vi "Position module.vi"(8 "error in (no error)":errorcluster) -> (0 "error out":errorcluster)   [LabVIEW 2016]
uses:
  General/Controls/data modes.ctl
  DAQ/Controls/DAQ queue.ctl
  DAQ/Controls/Queue states.ctl
  General/Controls/Queue modes.ctl
  Controls/Actuator fgv modes.ctl
  General/Controls/staus modes.ctl
  Controls/Command cluster.ctl
  Controls/Command list.ctl
  General/Controls/State control cluster.ctl
  General/Controls/States.ctl
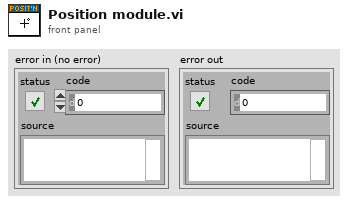
[diagram p1: front panel]
types:
  T1 = typedef "Queue modes.ctl" = enum16{"Initialise", "Destroy", "Get"}
  T2 = typedef "DAQ queue.ctl" = cluster{"Sate":T3, "Data":variant}
  T3 = typedef "Queue states.ctl" = enum16{"Shutdown", "Save data", "Record", "Read", "Setup", "Zero", "Connect", "Initialise"}
  T4 = typedef "data modes.ctl" = enum16{"Initalise", "Status", "Process", "Add load", "Add position"}
  T5 = cluster{"seconds since 1Jan1904":timestamp, "Numeric 2":dbl}[]
  T6 = typedef "References.ctl" = cluster{"Tab Control":refnum<vi>, "Logo 1":refnum<vi>, "Logo 2":refnum<vi>, "Connect Actuator":refnum<vi>, "LIVE DATA":refnum<vi>, "Speed":refnum<vi>, "Home position":refnum<vi>, "Limit position":refnum<vi>, "Trigger":refnum<vi>, "Current position":refnum<vi>, "Connect Camera":refnum<vi>, "TEST DATA":refnum<vi>, "LIVE DATA Force":refnum<vi>, "Connect DAQ":refnum<vi>, "Initialised":refnum<vi>, "Test":refnum<vi>}
  T7 = typedef "UEs.ctl" = cluster{"Read position":refnum<user-event>, "Check home":refnum<user-event>, "Record":refnum<user-event>, "Abort controller":refnum<user-event>, "Remote test":refnum<user-event>, "Test setup":refnum<user-event>, "Conditional wait":refnum<user-event>, "Abort move":refnum<user-event>, "Wait done":refnum<user-event>, "Send trigger":refnum<user-event>, "Initalising":refnum<user-event>, "Initalisation complete":refnum<user-event>}
  T8 = typedef "staus modes.ctl" = enum16{"Status", "Testing", "Webcam", "DAQ", "Actuator", "Initialise"}
  T9 = typedef "Actuator fgv modes.ctl" = enum16{"Initalise", "COM", "Limit", "Speed", "Home", "Get"}
  T10 = typedef "State control cluster.ctl" = cluster{"State":T11, "Data":variant}
  T11 = typedef "States.ctl" = enum16{"Initialise", "Actuator connection", "Get info", "Send command", "Load method", "Run method", "Save test", "Setup", "Shutdown"}
  T12 = typedef "Command cluster.ctl" = cluster{"Command":T13, "data":variant}
  T13 = typedef "Command list.ctl" = enum16{"", "£nabort", "getaxisno", "£getserialno", "£nidentify", "&&£setnlimit", "&£nm", "&£snv", "&£speed", "£np", "£ncal"}
  T14 = typedef "Default settings.ctl" = cluster{"COM port":refnum<visa-resource-name>, "Home pos":dbl, "Speed":dbl, "Limit stop":dbl}
  T15 = cluster{"seconds since 1Jan1904":timestamp, "Numeric 2":dbl}
  T16 = typedef "Test settings.ctl" = cluster{"Speed (mm/s)":dbl, "Position limit":bool, "Position limit (mm)":dbl, "Load limit":bool, "Load limit (N)":dbl, "No. of repeats":u16, "Test identifier":string, "Time wait":bool, "Wait time (s)":dbl, "Trigger wait":bool, "Send trigger":bool, "Test notes":string, "Snap intervals":bool, "Time interval (s)":dbl}
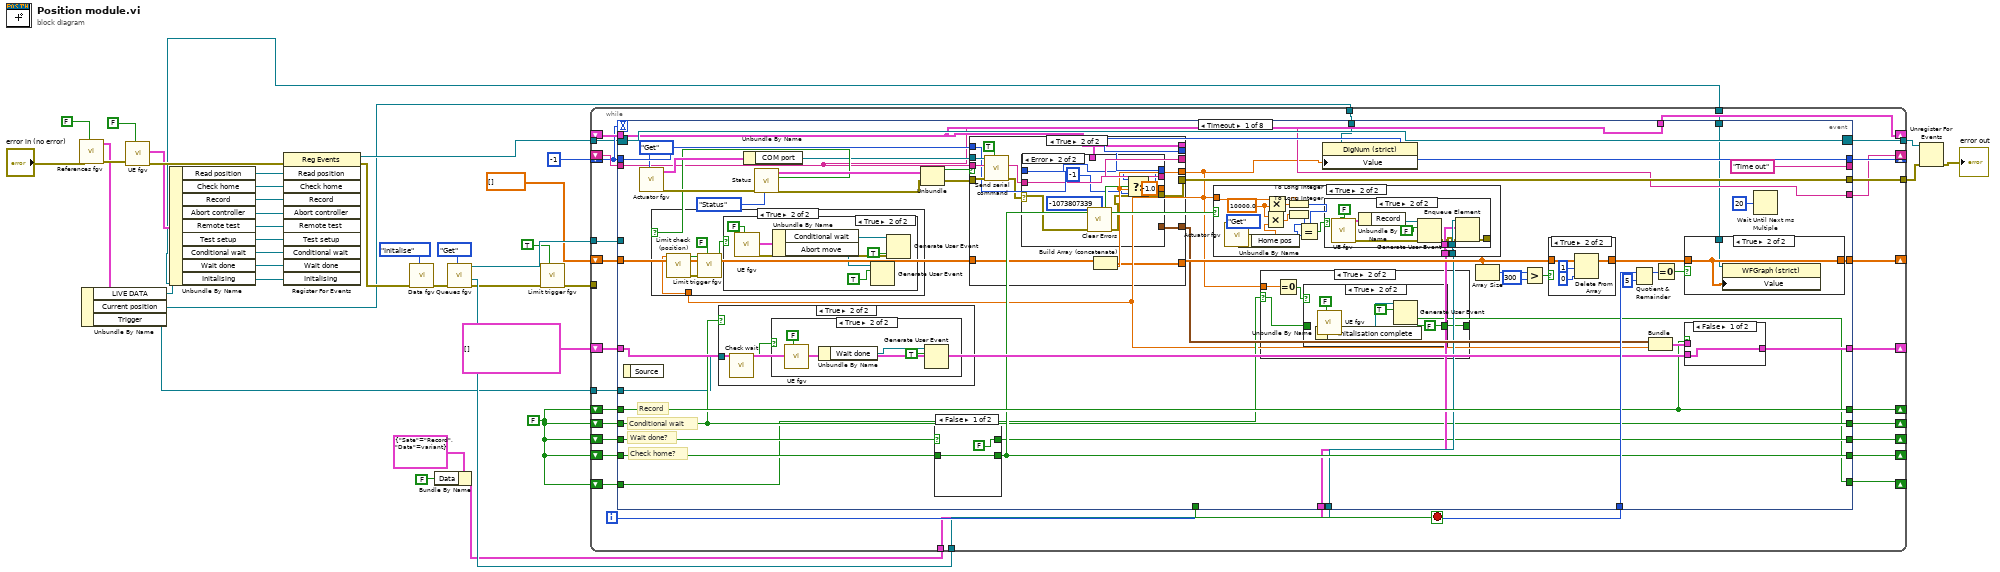
[diagram p0: block diagram]
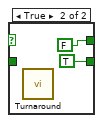
[diagram p10: hidden frame]
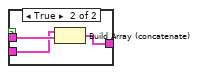
[diagram p11: hidden frame]
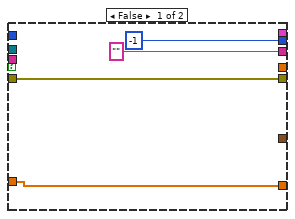
[diagram p14: hidden frame]
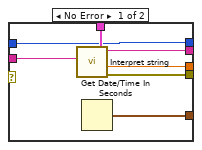
[diagram p15: hidden frame]
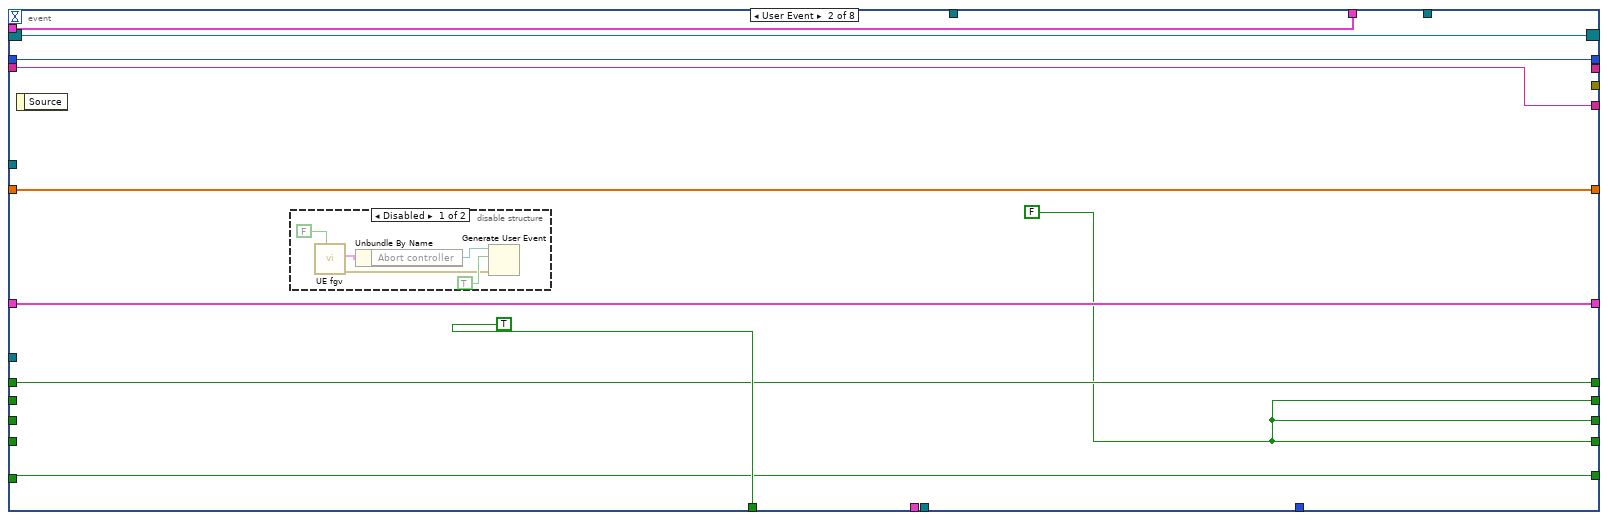
[diagram p16: hidden frame]
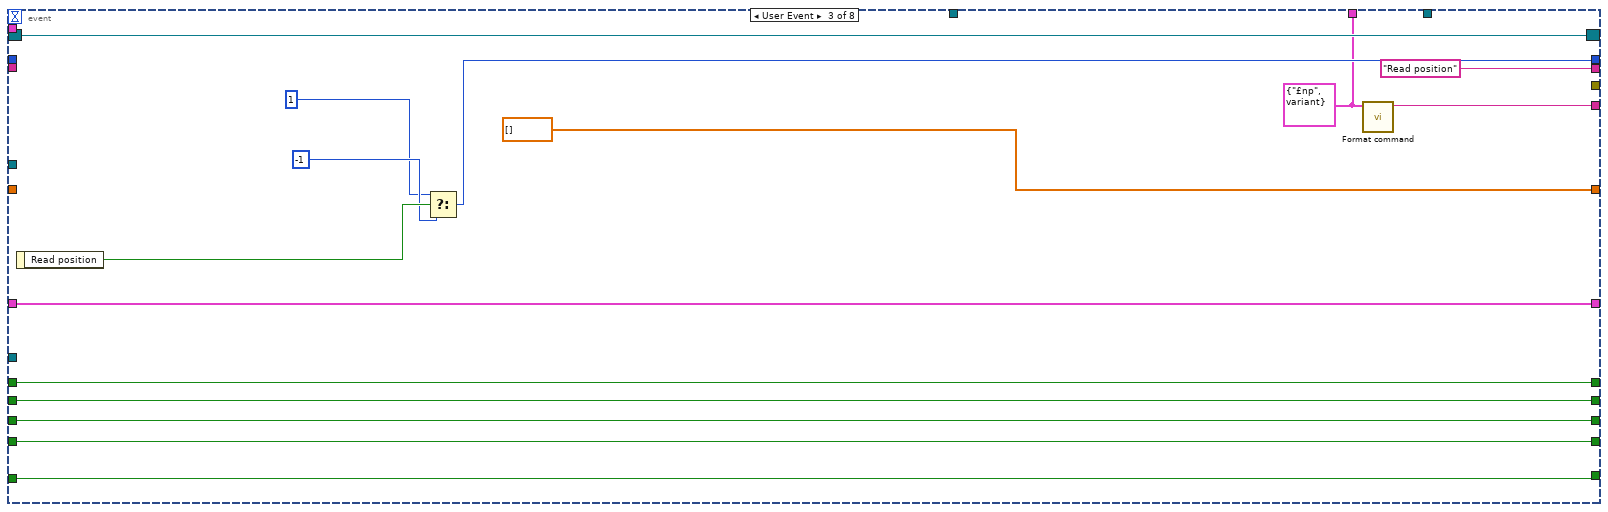
[diagram p18: hidden frame]
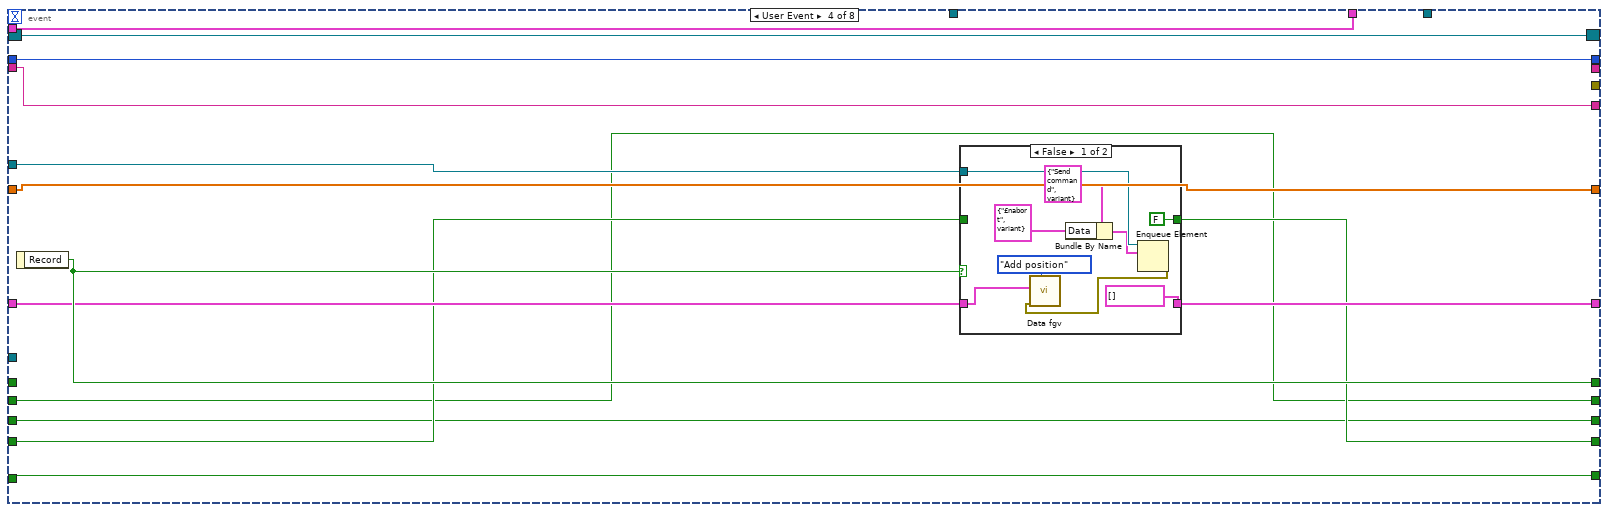
[diagram p19: hidden frame]
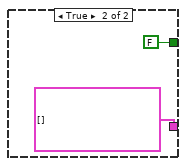
[diagram p20: hidden frame]
diagram:
  w1 = FALSE ("Record")
  n1 = call "References fgv.vi"("Set?"=FALSE, "error in (no error)"="error in (no error)") -> ("error out"=w8:errorcluster, "Cluster"=w6:T6)  [unwired: 8 in]
  n2 = Unbundle By Name(w6) -> ("LIVE DATA"=w3:refnum<vi>, "Current position"=w4:refnum<vi>, "Trigger"=w5:refnum<vi>)
  n3 = call "UE fgv.vi"("Set?"=FALSE, "error in (no error)"=w8) -> ("error out"=w33:errorcluster, "UEs"=w30:T7)  [unwired: 7 in, 1 out]
  n4 = Unbundle By Name(w30) -> ("Read position"=w19:refnum<user-event>, "Check home"=w20:refnum<user-event>, "Record"=w21:refnum<user-event>, "Abort controller"=w22:refnum<user-event>, "Remote test"=w23:refnum<user-event>, "Test setup"=w24:refnum<user-event>, "Conditional wait"=w26:refnum<user-event>, "Wait done"=w27:refnum<user-event>, "Initalising"=w2:refnum<user-event>)
  n5 = register-events(error in=w33, w19, w20, w21, w22, w23, w24, w26, w27, w2) -> (reference out=w25:refnum<event-registration>, error out=w32:errorcluster)  [unwired: 1 in]
  n6 = call "Data fgv.vi"("Modes"=data_modes."Initalise", "error in (no error)"=w32) -> ("error out"=w11:errorcluster)  [unwired: 5 in, 4 out]
  n7 = Bundle By Name(cluster=T2 {"Sate"=enum."Record", "Data"=variant} ("element"), "Data"=FALSE) -> (w18:T2)
  n8 = call "Queues fgv.vi"("Modes"=Queue_modes."Get", "error in (no error)"=w11) -> ("error in (no error) 2"=w10:errorcluster, "DAQ"=w39:refnum<queue>, "Ivium"=w38:refnum<queue>)  [unwired: 6 in, 1 out]
  n9 = call "Limit trigger fgv.vi"("Reset"=TRUE, "error in (no error)"=w10) -> ("error out"=w28:errorcluster)  [unwired: 8 in, 1 out]
  n10 = while {
    tunnel: [w69] -> w35
    tunnel: w25 -> [w53]
    shift-right: [w67] -> _
    shift-left: -1 -> [w66]
    shift-right: [w64] -> _
    shift-left: dbl[] [] -> [w65]
    shift-right: [w62] -> _
    shift-left: w1 -> [w61]
    shift-right: [w59] -> _
    shift-left: T5 [] -> [w60]
    tunnel: w39 -> [w58]
    tunnel: w18 -> [w57]
    tunnel: w38 -> [w56]
    shift-right: [w54] -> _
    shift-left: w1 -> [w55]
    shift-right: [w51] -> _
    shift-left: w1 -> [w52]
    shift-right: [w49] -> _
    shift-left: w1 -> [w50]
    tunnel: [w48] -> _
    tunnel: w28 -> [w48]
    tunnel: w5 -> [w47]
    tunnel: [w46] -> w34
    shift-right: [w45] -> _
    shift-left: _ -> [w70]
    shift-right: [w44] -> _
    shift-left: _ -> [w71]
    tunnel: w4 -> [w43]
    tunnel: w3 -> [w42]
    shift-right: [w40] -> _
    shift-left: w1 -> [w41]
    i -> [w63]
    stop <- w68 stop-if-true
    n11 = event shown="[0] Timeout" {
      selector: w53 -> [w116 w227 w244 w261 w280 w298 w315 w326]
      dyn-events: [w116 w227 w244 w261 w280 w298 w315 w326] -> w46
      timeout: w66 -> [_ _ _ _ _ _ _ _]
      tunnel: w71 -> [w77 w220 _ w250 w275 w286 w309 w322]
      tunnel: w70 -> [w78 w221 _ w251 w276 w287 w310 w323]
      tunnel: [w117 _ _ _ _ _ _ _] -> w69
      tunnel: [_ TRUE _ _ _ _ _ _] -> w68
      tunnel: [w113 w226 w245 w262 w281 w299 w316 w327] -> w67
      tunnel: w66 -> [w114 w226 _ w262 w281 w299 w316 w327]
      tunnel: w65 -> [w107 w225 _ w257 w282 w300 w317 w328]
      tunnel: [w84 w225 dbl[] [] w257 w282 w300 w317 w328] -> w64
      tunnel: w63 -> [w102 _ _ _ _ _ _ _]
      tunnel: [w94 w223 w241 w260 w279 w297 w314 w325] -> w62
      tunnel: w61 -> [w94 w223 w241 _ w279 w297 w314 w325]
      tunnel: w60 -> [w95 w224 w242 w259 w283 w301 w318 w329]
      tunnel: [w93 w224 w242 w258 w283 w301 w318 w329] -> w59
      tunnel: w58 -> [w90 _ _ _ _ _ _ _]
      tunnel: w57 -> [w89 _ _ _ _ _ _ _]
      tunnel: w56 -> [_ _ _ w256 _ _ _ _]
      tunnel: w55 -> [w92 _ w240 w255 _ w296 w313 w324]
      tunnel: [w91 w222 w240 w254 w284 w296 w313 w324] -> w54
      tunnel: w52 -> [w87 _ w239 w253 w278 _ _ w321]
      tunnel: [w87 w222 w239 w253 w278 TRUE ("Record") FALSE ("Record") w321] -> w51
      tunnel: w50 -> [w83 _ w238 w252 w277 _ _ w320]
      tunnel: [w82 w222 w238 w252 w277 FALSE ("Record") TRUE ("Record") w320] -> w49
      tunnel: w47 -> [w81 _ _ _ _ _ _ _]
      tunnel: ["Time out" _ "Read position" _ _ _ _ _] -> _
      tunnel: [w78 w221 w236 w251 w276 w287 w310 w323] -> w45
      tunnel: [w77 w220 w235 w250 w275 w286 w309 w322] -> w44
      tunnel: w43 -> [w76 _ _ _ _ _ _ _]
      tunnel: w42 -> [w75 _ _ _ _ _ _ _]
      tunnel: w41 -> [w74 w219 w234 w249 w274 w285 w308 _]
      tunnel: [w72 w219 w234 w249 w274 w285 w308 TRUE ("Record")] -> w40
      event Timeout {
        # "Wait done?"
        # "Record"
        # "Conditional wait"
        # "Check home?"
        n12 = event-data() -> ()  [unwired: 1 in, 1 out]
        n13 = call "Actuator fgv.vi"("Enum"=Actuator_fgv_modes."Get") -> ("error out"=w112:errorcluster, "Cluster out"=w115:T14)  [unwired: 9 in]
        n14 = case shown="True" w87 {
          tunnel: w81 -> [_ w141]
          frame False {
          }
          frame True {
            n15 = call "Check wait.vi"("Trigger"=w141) -> ("Wait done?"=w142:bool)  [unwired: 10 in]
            n16 = case shown="True" w142 {
              frame False {
              }
              frame True {
                n17 = call "UE fgv.vi"("Set?"=FALSE) -> ("UEs"=w146:T7)  [unwired: 8 in, 2 out]
                n18 = Unbundle By Name(w146) -> ("Wait done"=w145:refnum<user-event>)
                n19 = Generate User Event(user event=w145, event data cluster=TRUE ("event data")) -> ()  [unwired: 2 in, 2 out]
              }
            }
          }
        }
        n20 = Unbundle By Name(w115) -> ("COM port"=w79:refnum<visa-resource-name>)
        n21 = call "Status.vi"("Mode"=staus_modes."Status", "error in (no error)"=w112) -> ("error out"=w111:errorcluster, "Testing"=w86:bool, "Connections"=w110:cluster{"Data":bool, "Data":bool, "Data":bool})  [unwired: 7 in]
        n22 = Unbundle(w110) -> ("Data"=w109:bool)  [unwired: 2 out]
        n23 = case shown="False" w83 {
          tunnel: w92 -> [w169 _]
          tunnel: [w169 TRUE ("Record")] -> w91
          tunnel: [FALSE ("Record") FALSE ("Record")] -> w82
          frame False {
          }
          frame True {
            n24 = call "Turnaround.vi"() -> ()  [unwired: 11 in, 1 out]
          }
        }
        n25 = case shown="True" w109 {
          tunnel: w77 -> [_ w202]
          tunnel: w78 -> [_ w201]
          tunnel: [w186 w199] -> w117
          tunnel: [_ w191] -> w73
          tunnel: ["" ("String 2") w197] -> _
          tunnel: w111 -> [w186 w196]
          tunnel: w79 -> [_ w195]
          tunnel: w114 -> [_ w194]
          tunnel: [-1 w193] -> w113
          tunnel: w107 -> [w184 w192]
          tunnel: [w184 w190] -> w100
          tunnel: [_ w189] -> w97
          frame False {
          }
          frame True {
            n26 = call "Send serial command.vi"("Read?"=TRUE, "error IO"=w196, "Send string"=w202, "VISA resource name out"=w195) -> ("error out"=w188:errorcluster, "read string"=w200:string)  [unwired: 5 in, 1 out]
            n27 = case shown="Error" w188 {
              selector: w188 -> [_ w216]
              tunnel: w201 -> [w209 _]
              tunnel: w200 -> [w208 w218]
              tunnel: [w207 w215] -> w199
              tunnel: [w206 -1.0 ("Numeric 2")] -> w191
              tunnel: [w205 w218] -> w197
              tunnel: w194 -> [w204 w211]
              tunnel: [w204 w212] -> w193
              tunnel: [w203 _] -> w189
              frame No Error {
                n28 = call "Interpret string.vi"("String"=w208, "Cluster"=w209) -> ("error out"=w207:errorcluster, "Numeric 2"=w206:dbl, "String 2"=w205:string)  [unwired: 6 in, 1 out]
                n29 = Get Date/Time In Seconds() -> (seconds since 1Jan1904=w203:timestamp)
              }
              frame Error {
                n30 = call <vilib>:"Clear Errors.vi"("error in (no error)"=w216, "specific error code to clear (0: all)"=-1073807339) -> ("error out"=w215:errorcluster, "specific error cleared?"=w214:bool)  [unwired: 4 in]
                n31 = Select(t=w211, s=w214, f=-1) -> (s? t:f=w212:i32)
              }
            }
            n32 = Build Array (concatenate)(w192, w191) -> (w190:dbl[])
          }
        }
        n33 = case shown="True" w86 {
          tunnel: w73 -> [_ w133]
          frame False {
          }
          frame True {
            n34 = call "Limit check (position).vi"("position"=w133) -> ("error out"=w132:errorcluster, "Limit?"=w131:bool)  [unwired: 9 in]
            n35 = call "Limit trigger fgv.vi"("Reset"=FALSE, "error in (no error)"=w132, "Set"=w131) -> ("Limit trigger"=w130:bool)  [unwired: 7 in, 1 out]
            n36 = case shown="True" w130 {
              frame False {
              }
              frame True {
                n37 = call "UE fgv.vi"("Set?"=FALSE) -> ("error out"=w140:errorcluster, "UEs"=w139:T7)  [unwired: 8 in, 1 out]
                n38 = Unbundle By Name(w139) -> ("Conditional wait"=w138:refnum<user-event>, "Abort move"=w136:refnum<user-event>)
                n39 = Generate User Event(user event=w136, event data cluster=TRUE ("event data")) -> ()  [unwired: 2 in, 2 out]
                n40 = Generate User Event(user event=w138, event data cluster=TRUE ("event data"), error in=w140) -> ()  [unwired: 1 in, 2 out]
              }
            }
          }
        }
        n41 = case shown="True" w91 {
          tunnel: w73 -> [_ w154]
          tunnel: w90 -> [_ w156]
          tunnel: w89 -> [_ w155]
          frame False {
          }
          frame True {
            w152 = 10000.0 ("y")
            n42 = call "Actuator fgv.vi"("Enum"=Actuator_fgv_modes."Get") -> ("Cluster out"=w157:T14)  [unwired: 9 in, 1 out]
            n43 = Unbundle By Name(w157) -> ("Home pos"=w153:dbl)
            n44 = Multiply(x=w152, y=w153) -> (x*y=w150:dbl)
            n45 = Multiply(x=w154, y=w152) -> (x*y=w151:dbl)
            n46 = To Long Integer(number=w151) -> (32bit integer=w148:i32)
            n47 = To Long Integer(number=w150) -> (32bit integer=w147:i32)
            n48 = Equal?(x=w148, y=w147) -> (x = y?=w149:bool)
            n49 = case shown="True" w149 {
              tunnel: w156 -> [_ w166]
              tunnel: w155 -> [_ w165]
              tunnel: [_ w159] -> _
              frame False {
              }
              frame True {
                n50 = call "UE fgv.vi"("Set?"=FALSE) -> ("error out"=w160:errorcluster, "UEs"=w164:T7)  [unwired: 8 in, 1 out]
                n51 = Unbundle By Name(w164) -> ("Record"=w162:refnum<user-event>)
                n52 = Generate User Event(user event=w162, event data cluster=FALSE ("event data"), error in=w160) -> (error out=w161:errorcluster)  [unwired: 1 in, 1 out]
                n53 = Enqueue Element(queue=w166, element=w165, error in (no error)=w161) -> (error out=w159:errorcluster)  [unwired: 1 in, 2 out]
              }
            }
          }
        }
        n54 = case shown="True" w74 {
          selector: w74 -> [w118 w119]
          tunnel: w73 -> [_ w122]
          tunnel: [w118 w120] -> w72
          frame False {
          }
          frame True {
            n55 = Equal To 0?(x=w122) -> (x = 0?=w121:bool)
            n56 = case shown="True" w121 {
              tunnel: [w123 FALSE] -> w120
              tunnel: w119 -> [w123 _]
              frame False {
              }
              frame True {
                n57 = call "UE fgv.vi"("Set?"=FALSE) -> ("UEs"=w127:T7)  [unwired: 8 in, 2 out]
                n58 = Unbundle By Name(w127) -> ("Initalisation complete"=w125:refnum<user-event>)
                n59 = Generate User Event(user event=w125, event data cluster=TRUE ("event data")) -> ()  [unwired: 2 in, 2 out]
              }
            }
          }
        }
        n60 = property class="DigNum (strict)"(reference=w76, "Value"=w73) -> ()  [unwired: 1 in, 2 out]
        n61 = Array Size(array=w100) -> (size(s)=w106:i32)
        n62 = Greater?(x=w106, y=300) -> (0:w104:bool)
        n63 = case shown="True" w104 {
          tunnel: w100 -> [w179 w183]
          tunnel: [w179 w180] -> w85
          frame False {
          }
          frame True {
            n64 = Delete From Array(array=w183, length=1, index=0) -> (array with subset deleted=w180:dbl[])  [unwired: 1 out]
          }
        }
        n65 = Quotient & Remainder(x=w102, y=5 ("x")) -> (x-y*floor(x/y)=w99:i32)  [unwired: 1 out]
        n66 = Bundle("seconds since 1Jan1904"=w97, "Numeric 2"=w73) -> (w96:T15)  [unwired: 1 in]
        n67 = Equal To 0?(x=w99) -> (x = 0?=w98:bool)
        n68 = case shown="False" w94 {
          tunnel: w96 -> [_ w175]
          tunnel: w95 -> [w172 w174]
          tunnel: [w172 w173] -> w93
          frame False {
          }
          frame True {
            n69 = Build Array (concatenate)(w174, w175) -> (w173:T5)
          }
        }
        n70 = case shown="True" w98 {
          tunnel: w85 -> [w176 w178]
          tunnel: [w176 w178] -> w84
          tunnel: w75 -> [_ w177]
          frame False {
          }
          frame True {
            n71 = property class="WFGraph (strict)"(reference=w177, "Value"=w178) -> ()  [unwired: 1 in, 2 out]
          }
        }
        n72 = Wait Until Next ms Multiple(millisecond multiple=u32 20) -> ()  [unwired: 1 out]
      }
      event User Event {
        w222 = FALSE ("Record")
        n73 = event-data() -> ()  [unwired: 1 in, 1 out]
        n74 = disable-structure shown="Disabled" {
          frame Disabled {
            n75 = call "UE fgv.vi"("Set?"=FALSE) -> ("error out"=w231:errorcluster, "UEs"=w233:T7)  [unwired: 8 in, 1 out]
            n76 = Unbundle By Name(w233) -> ("Abort controller"=w229:refnum<user-event>)
            n77 = Generate User Event(user event=w229, event data cluster=TRUE ("Discard?"), error in=w231) -> ()  [unwired: 1 in, 2 out]
          }
          frame Enabled {
          }
        }
      }
      event User Event {
        w236 = T12 {"Command"=enum."£np", "data"=variant} ("Cluster")
        n78 = event-data() -> ("Read position"=w248:bool)  [unwired: 1 in]
        n79 = Select(t=1, s=w248, f=-1) -> (s? t:f=w245:i32)
        n80 = call "Format command.vi"("Cluster"=w236) -> ("String"=w235:string)  [unwired: 9 in, 1 out]
      }
      event User Event {
        n81 = event-data() -> ("Record"=w260:bool)  [unwired: 1 in]
        n82 = case shown="False" w260 {
          tunnel: w259 -> [w269 _]
          tunnel: [T5 [] T5 []] -> w258
          tunnel: w256 -> [w268 _]
          tunnel: w255 -> [_ _]
          tunnel: [FALSE FALSE] -> w254
          frame False {
            n83 = Bundle By Name(cluster=T10 {"State"=enum."Send command", "Data"=variant} ("element"), "Data"=T12 {"Command"=enum."£nabort", "data"=variant} ("Cluster")) -> (w265:T10)
            n84 = Enqueue Element(queue=w268, element=w265) -> (error out=w264:errorcluster)  [unwired: 2 in, 2 out]
            n85 = call "Data fgv.vi"("Modes"=data_modes."Add position", "error in (no error)"=w264, "Data"=w269) -> ()  [unwired: 4 in, 5 out]
          }
          frame True {
          }
        }
      }
      event User Event {
        n86 = event-data() -> ("Check home"=w284:bool)  [unwired: 1 in]
      }
      event User Event {
        n87 = event-data() -> ()  [unwired: 1 in, 1 out]
        n88 = call "Timer.vi"("Reset"=TRUE) -> ("error out"=w292:errorcluster)  [unwired: 9 in, 1 out]
        n89 = call "Test settings fgv.vi"("Set?"=FALSE, "error in (no error)"=w292) -> ("error out"=w288:errorcluster, "Test settings out"=w290:T16)  [unwired: 7 in, 1 out]
        n90 = Unbundle By Name(w290) -> ("Send trigger"=w289:bool)
        n91 = case shown="True" w289 {
          tunnel: w288 -> [_ w302]
          frame False {
          }
          frame True {
            n92 = call "UE fgv.vi"("Set?"=FALSE, "error in (no error)"=w302) -> ("error out"=w303:errorcluster, "UEs"=w306:T7)  [unwired: 7 in, 1 out]
            n93 = Unbundle By Name(w306) -> ("Send trigger"=w305:refnum<user-event>)
            n94 = Generate User Event(user event=w305, event data cluster=TRUE ("event data"), error in=w303) -> ()  [unwired: 1 in, 2 out]
          }
        }
      }
      event User Event {
        n95 = event-data() -> ()  [unwired: 1 in, 1 out]
      }
      event User Event {
        (unwired) FALSE ("Record")
        n96 = event-data() -> ()  [unwired: 1 in, 1 out]
      }
    }
  }
  n97 = Unregister For Events(event registration refnum=w34, error in=w35) -> (error out=→"error out":errorcluster)
